vi "parse-AI-string.vi"(9 "read buffer in":string=">+028.20+888888+888888+888888+888888+888888+888888", 11 "Analog Data":T1) -> (1 "csv":string, 3 "Analog Data Out":T1)   [LabVIEW 2020]
uses:
  <vilib>/regexp/Match Regular Expression.xnode
  controls/depreciated/analog-data-cluster.ctl
panel:
  out "result string 3":string
  out "result string 2":string
  out "result string":string
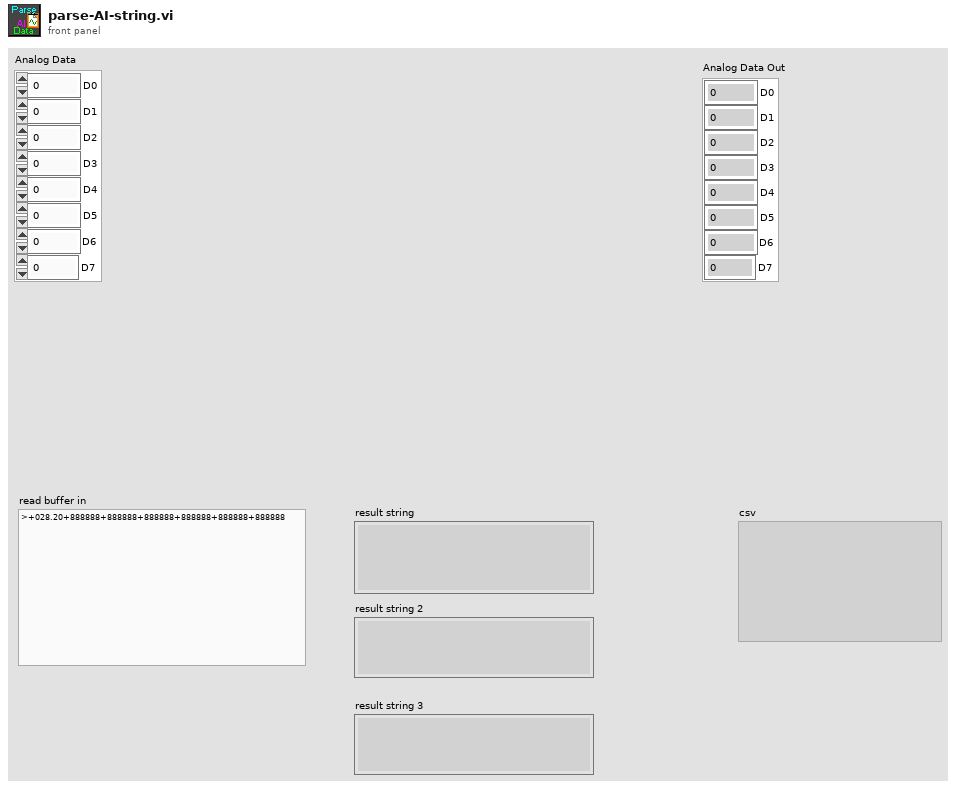
[diagram p1: front panel]
types:
  T1 = typedef "analog-data-cluster.ctl" = cluster{"D0":dbl, "D1":dbl, "D2":dbl, "D3":dbl, "D4":dbl, "D5":dbl, "D6":dbl, "D7":dbl}
  T2 = cluster{"Analog Data[0]":dbl, "Analog Data[1]":dbl, "Analog Data[2]":dbl, "Analog Data[3]":dbl, "Analog Data[4]":dbl, "Analog Data[5]":dbl, "Analog Data[6]":dbl, "Analog Data[7]":dbl, "Analog Data[8]":dbl}
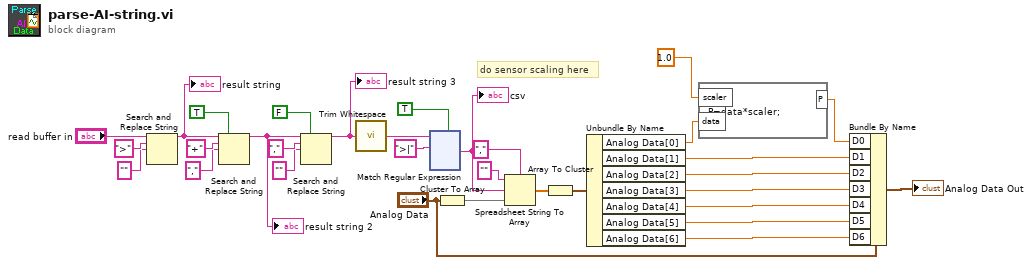
[diagram p0: block diagram]
diagram:
  # "do sensor scaling here"
  n1 = Search and Replace String(input string="read buffer in", search string=">", replace string="" ("replace string (\"\")")) -> (result string=w17:string)  [unwired: 5 in, 3 out]
  "result string" <- w17
  n2 = Search and Replace String(replace all?=TRUE ("replace all? (F)"), input string=w17, search string="+", replace string="," ("replace string (\"\")")) -> (result string=w11:string)  [unwired: 4 in, 3 out]
  "result string 2" <- w11
  n3 = Search and Replace String(replace all?=FALSE ("replace all? (F)"), input string=w11, search string=",", replace string="" ("replace string (\"\")")) -> (result string=w5:string)  [unwired: 4 in, 3 out]
  "result string 3" <- w5
  n4 = call <vilib>:"Trim Whitespace.vi"("string"=w5) -> ("trimmed string"=w6:string)  [unwired: 1 in]
  n5 = xnode "Match Regular Expression"("input string"=w6, "regular expression"=">|", "multiline? (F)"=TRUE) -> ("after match"=w4:string)  [unwired: 3 in, 4 out]
  "csv" <- w4
  n6 = Cluster To Array(cluster="Analog Data") -> (array=w29:dbl[])
  n7 = Spreadsheet String To Array(delimiter (Tab)=",", format string="", spreadsheet string=w4, array type (2D Dbl)=w29) -> (array=w30:dbl[])
  n8 = Array To Cluster(array=w30) -> (cluster=w31:T2)
  n9 = Unbundle By Name(w31) -> ("Analog Data[0]"=w3:dbl, "Analog Data[1]"=w27:dbl, "Analog Data[2]"=w26:dbl, "Analog Data[3]"=w25:dbl, "Analog Data[4]"=w24:dbl, "Analog Data[5]"=w23:dbl, "Analog Data[6]"=w22:dbl)
  n10 = formula code="P=data*scaler;"("data"=w3, "scaler"=1.0 ("input variable")) -> ("P"=w1:dbl)
  n11 = Bundle By Name(cluster="Analog Data", "D0"=w1, "D1"=w27, "D2"=w26, "D3"=w25, "D4"=w24, "D5"=w23, "D6"=w22) -> (→"Analog Data Out":T1)
